vi "Drive_Globals.vi"() -> ()   [LabVIEW 2019]
uses:
  Drive_Cluster.ctl
  MARS-2020/mOS_XIII/MoS_XIII/Subsystems/Drive/Drive_States.ctl
panel:
  in  "Drive_IMU":string="Drive_IMU"
  in  "Drive_Left_Master":string="Drive_Left_Master"
  in  "Drive_Left_Slave":string="Drive_Left_Slave"
  in  "Drive_Right_Slave":string="Drive_Right_Slave"
  in  "Drive_Right_Master":string="Drive_Right_Master"
  in  "Drive_Execute_Notifier":refnum<notifier>
  in  "Drive_Set_Notifier":refnum<notifier>
  in  "Drive_Execute_Ref":string="Drive_Execute_Ref"
  in  "Drive_Set_Ref":string="Drive_Set_Ref"
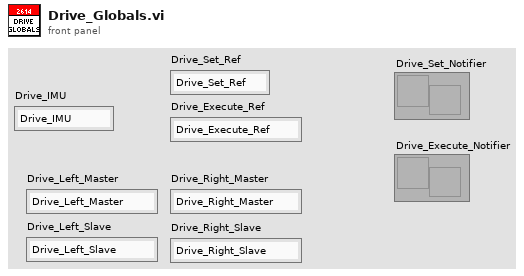
[diagram p1: front panel]
diagram:
